vi "QT_MovieOpen.vi"(2 "File Settings":T1 {"Dialogs" format="%.0b"}, 5 "error in (no error)":errorcluster, 8 "Private":T3) -> (14 "QT Ref Out":T2, 16 "Movie info":T4 {"Tracks"."Rate" format="%.2f"}, 19 "error out":errorcluster)   [LabVIEW 2024]
uses:
  <userlib>/ImageProcessing/QTLIB_2595_LV86/QT_Selector.ctl
  <userlib>/ImageProcessing/QTLIB_2595_LV86/QT_Track.ctl
  <userlib>/ImageProcessing/QTLIB_2595_LV86/QT_MovieInfo.ctl
  <userlib>/ImageProcessing/QTLIB_2595_LV86/QT_Private.ctl
  <userlib>/ImageProcessing/QTLIB_2595_LV86/QT_Ref.ctl
  <userlib>/ImageProcessing/QTLIB_2595_LV86/QT_File.ctl
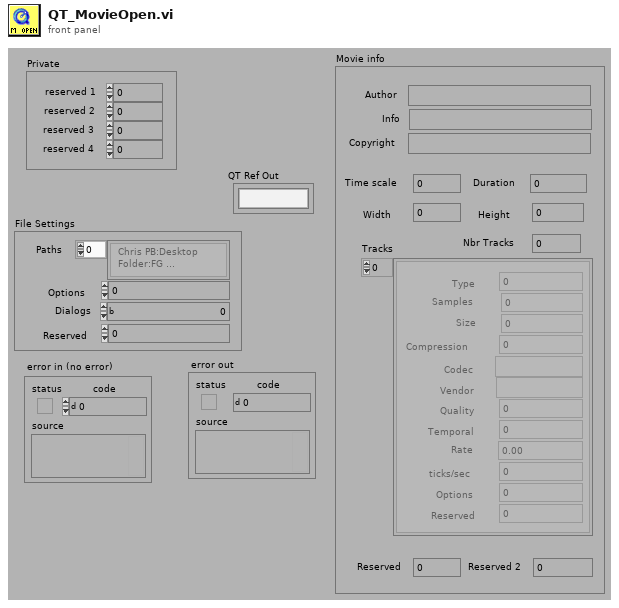
[diagram p1: front panel]
types:
  T1 = typedef "QT_File.ctl" = cluster{"Paths":string[], "Options":i32, "Dialogs":u32, "Reserved":i32}
  T2 = typedef "QT_Ref.ctl" = refnum<k1>
  T3 = typedef "QT_Private.ctl" = cluster{"reserved 1":i32, "reserved 2":i32, "reserved 3":i32, "reserved 4":i32}
  T4 = typedef "QT_MovieInfo.ctl" = cluster{"Author":string, "Info":string, "Copyright":string, "Time scale":i32, "Duration":i32, "Width":i32, "Height":i32, "Nbr Tracks":i32, "Tracks":T5[], "Reserved":i32, "Reserved 2":i32}
  T5 = typedef "QT_Track.ctl" = cluster{"Type":i32, "Samples":i32, "Size":i32, "Compression":i32, "Codec":string, "Vendor":string, "Quality":i32, "Temporal":i32, "Rate ":dbl, "ticks/sec":i32, "Options":i32, "Reserved":i32}
  T6 = typedef "QT_Selector.ctl" = enum32{"do nothing", "Get all Sources", "Get Source info", "Open Image", "Save Image to File", "Effect", "Close", "SG Grab", "Compress in Memory", "Decompress to Memory", "New Movie", "Open Movie", "Add Frame", "Get Frame", "Close Movie", "Get QT & CIN info", "SG init", "SG Close", "Open sound file", "Close sound file", "Read sound data", "Write sound data", "Import sound", "Export sound", "Add sound to movie", "Get sound from movie", "reserved", "reserved 1", "reserved 2"}
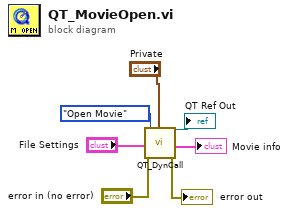
[diagram p0: block diagram]
diagram:
  n1 = call <userlib>:"QT_DynCall.vi"("error in (no error)"="error in (no error)", "Selector"=QT_Selector."Open Movie", "Private"="Private", "File Settings"="File Settings") -> ("QT Ref Out"=→"QT Ref Out":T2, "Movie info"=→"Movie info":T4, "error out"=→"error out":errorcluster)  [unwired: 8 in, 13 out]
